vi "Untitled 1.vi"(4 "?":refnum<vi>, 6 "CtlRef":refnum<vi>, 7 "Event Common Data":cluster{"Source":T1, "Type":T2, "Time":u32} {"Source" items=["LabVIEW UI"=0, "ActiveX"=1, "User Event"=25]}) -> ()   [LabVIEW 2013]
uses:
  <vilib>/event_ctls.llb/eventsource.ctl
  <vilib>/event_ctls.llb/lveventtype.ctl
panel:
  out "data":bool
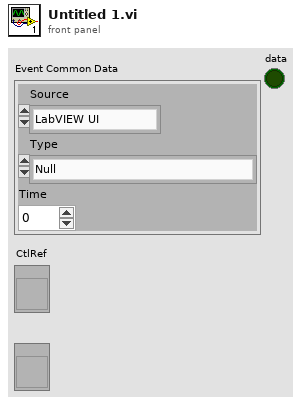
[diagram p1: front panel]
types:
  T1 = typedef "eventsource.ctl" = u32
  T2 = typedef "lveventtype.ctl" = enum32{"Null", "Timeout", "Annotation Menu Selection", "Annotation Menu Selection?", "App Instance Close", "App Instance Close?", "Autoscale Range Change", "Bookmark Info Change", "Cell Edit", "Cell Edit?", "Cursor Grab", "Cursor Grab?", "Cursor Menu Selection", "Cursor Menu Selection?", "Cursor Move", "Cursor Release", "Data Change", "Direction Change", "Display State Change", "Drag Ended", "Drag Enter", "Drag Leave", "Drag Over", "Drag Source Update", "Drag Starting", "Drag Starting?", "Drop", "Exec State Change", "Key Down", "Key Down?", "Key Repeat", "Key Repeat?", "Key Up", "Listbox Double Click", "Menu Activation?", "Menu Selection (App)", "Menu Selection? (App)", "Menu Selection (User)", "Mouse Down", "Mouse Down?", "Mouse Enter", "Mouse Leave", "Mouse Move", "Mouse Up", "Mouse Wheel", "NI Security User Change (App)", "Pane Size", "Panel Close", "Panel Close?", "Panel Resize", "Plot Attribute Change", "Scale Range Change", "Shortcut Menu Activation?", "Shortcut Menu Selection (App)", "Shortcut Menu Selection? (App)", "Shortcut Menu Selection (User)", "Tree Double Click", "Tree Drag", "Tree Drag?", "Tree Drop", "Tree Drop?", "Tree Item Close", "Tree Item Close?", "Tree Item Open", "Tree Item Open?", "User Event", "Value Change"}
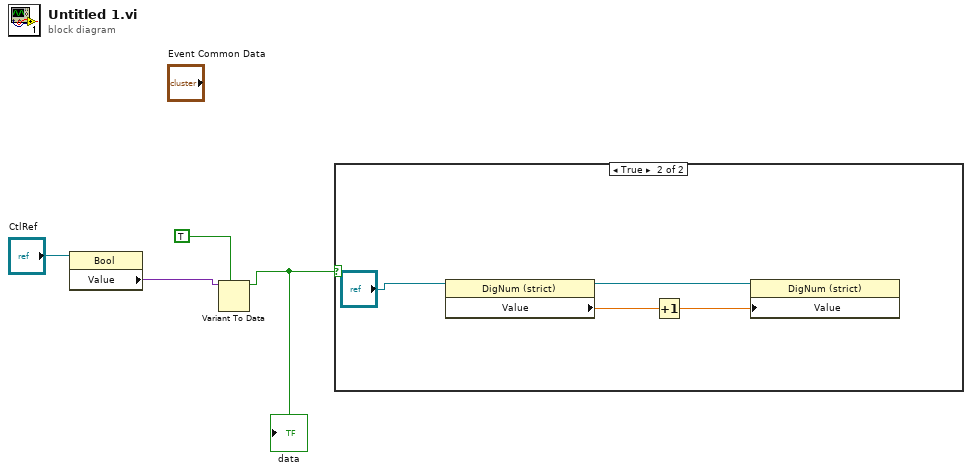
[diagram p0: block diagram]
diagram:
  n1 = property class="Bool"(reference="CtlRef") -> ("Value"=w3:variant)  [unwired: 1 in, 2 out]
  n2 = Variant To Data(type=TRUE, Variant=w3) -> (data=w2:bool)  [unwired: 1 in, 1 out]
  "data" <- w2
  n3 = case shown="True" w2 {
    frame False {
    }
    frame True {
      n4 = property class="DigNum (strict)"(reference="?") -> (reference out=w8:refnum<vi>, "Value"=w7:dbl)  [unwired: 1 in, 1 out]
      n5 = Increment(x=w7) -> (x+1=w6:dbl)
      n6 = property class="DigNum (strict)"(reference=w8, "Value"=w6) -> ()  [unwired: 1 in, 2 out]
    }
  }
